vi "GET XML.vi"(8 "error in (no error)":errorcluster, 11 "Domino Laser module Class in":refnum<class "Domino Laser module Class.lvclass">) -> (0 "error out":errorcluster, 2 "XML":string, 3 "Domino Laser module Class out":refnum<class "Domino Laser module Class.lvclass">)   [LabVIEW 2015, in "Domino LM.lvlib" / "Domino Laser module Class.lvclass"]
uses:
  CTRLS/Domino Laser module Class.lvclass
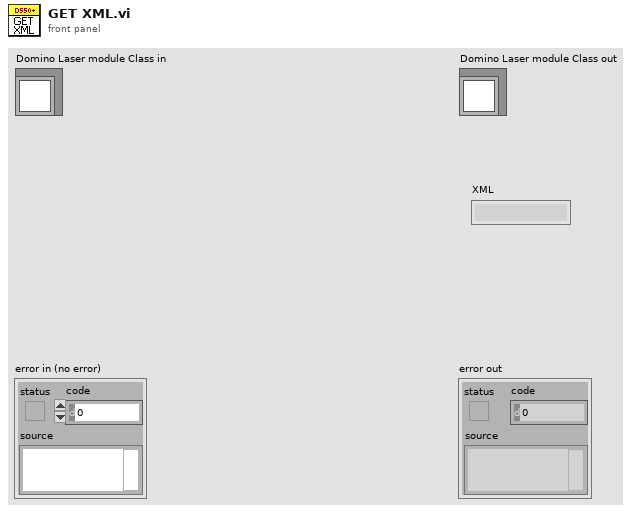
[diagram p1: front panel]
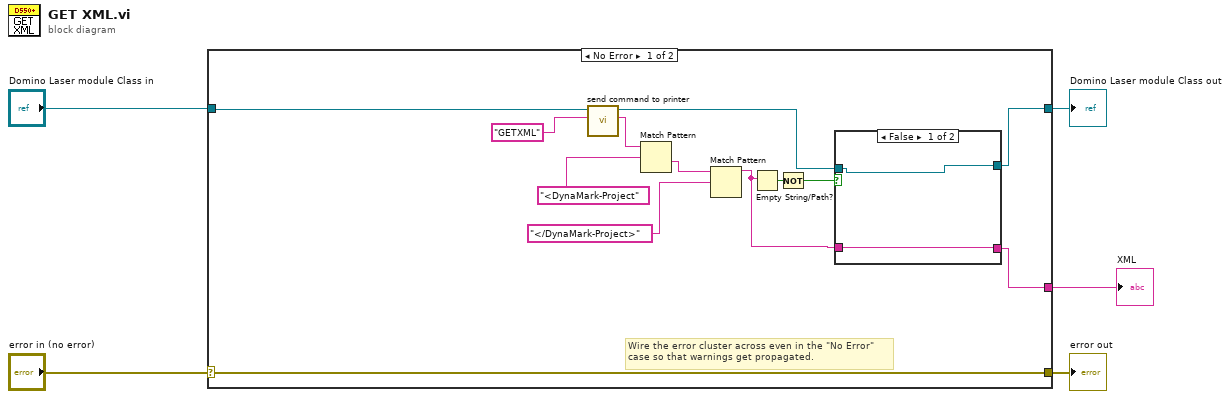
[diagram p0: block diagram]
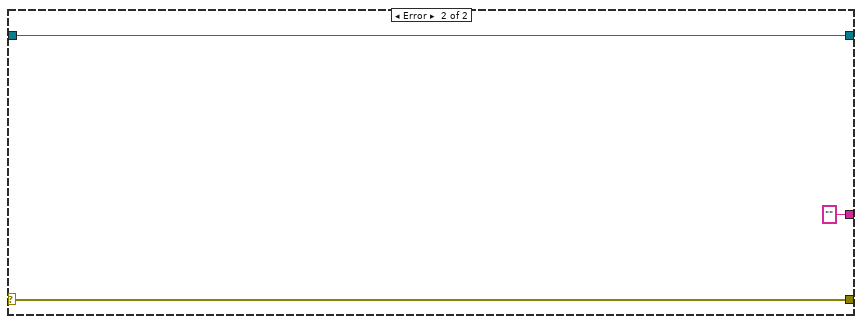
[diagram p3: hidden frame]
diagram:
  n1 = case shown="No Error" "error in (no error)" {
    selector: "error in (no error)" -> [w7 w25]
    tunnel: [w7 w25] -> w4
    tunnel: [w8 w24] -> w2
    tunnel: "Domino Laser module Class in" -> [w17 w24]
    tunnel: [w10 "" ("Recived message")] -> w1
    frame No Error {
      # "Wire the error cluster across even in the \"No Error\"\ncase so that warnings get propagated."
      n2 = call "send command to printer.vi"("command to be sent"="GETXML", "Domino Laser module Class in"=w17) -> ("Recived message"=w16:string, "Domino Laser module Class out"=w9:refnum<class "Domino Laser module Class.lvclass">)  [unwired: 6 in, 2 out]
      n3 = Match Pattern(string=w16, regular expression="<DynaMark-Project") -> (after substring=w14:string)  [unwired: 1 in, 3 out]
      n4 = Match Pattern(string=w14, regular expression="</DynaMark-Project>") -> (before substring=w6:string)  [unwired: 1 in, 3 out]
      n5 = Empty String/Path?(string/path=w6) -> (empty?=w12:bool)
      n6 = Not(x=w12) -> (.not. x?=w11:bool)
      n7 = case shown="False" w11 {
        tunnel: w6 -> [w19 w22]
        tunnel: [w19 w22] -> w10
        tunnel: w9 -> [w20 w21]
        tunnel: [w20 w21] -> w8
        frame False {
        }
        frame True {
        }
      }
    }
    frame Error {
    }
  }
  "error out" <- w4
  "Domino Laser module Class out" <- w2
  "XML" <- w1
